vi "Generate Error.vi"(0 "Optional String":string, 1 "Class":refnum<class>, 2 "Error Code":i32, 3 "Error/Warning":bool=TRUE) -> (6 "error out":errorcluster)   [LabVIEW 2026, in "TALOS.lvlib"]
doc: "This VI generates the custom error, given its number. If the optional flag \"Error/Warning\" is set to False, a warning is generated. The optional String gets appended at the end of the error message.\nIf a Class is given in input, its name will also be added to the error string."
uses:
  TALOS.lvlib
  <vilib>/Utility/error.llb/DialogType.ctl
  Ancestor/Ancestor/Ancestor.lvclass
  Ancestor/Ancestor/Ancestor.lvclass/Ancestor.ctl
  FGV/Error Memory/Error Memory Core.vi
  <vilib>/AdvancedString/Delimited String to 1D String Array.vi
  <vilib>/AdvancedString/Delimited String to 1D String Array (string).vi
  Circus Root Path.vi
  FGV/Error Memory/Error Crt Lvl checker.vi
  FGV/Error Memory/Error Memory Core.vi/40c8088d-b597-4017-91af-faa98e00292e.vi
  FGV/Error Memory/Error Memory Core.vi/d4a3ab98-063c-4e44-b43d-fbdcfe6c2be2.vi
  Global Memory.vi
  <vilib>/Utility/LVClass/Get LV Class Name.vi
  Is in Packed Library.vi
  TALOS Root path.vi
  Read CSV worksheet.vi
  Global Constants.vi
  <vilib>/Comparison/Equal/Equal Functor/Equal Functor.lvclass
  FGV/Error Memory/Error Memory.lvlib
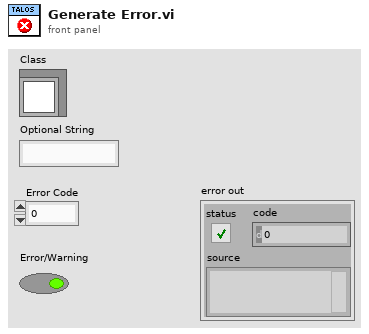
[diagram p1: front panel]
types:
  T1 = typedef "DialogType.ctl" = u16
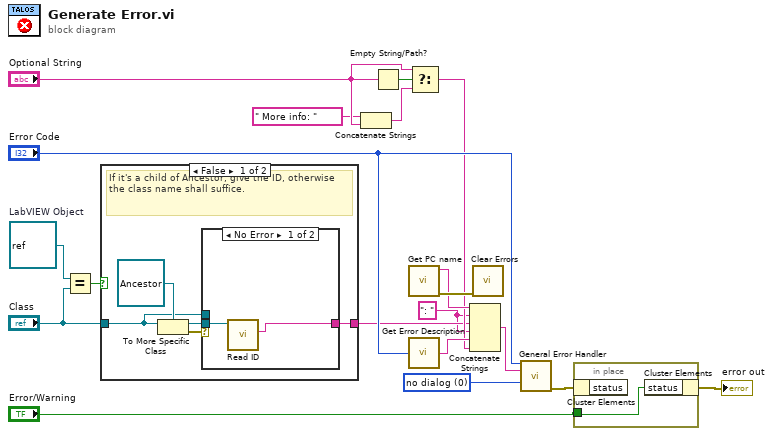
[diagram p0: block diagram]
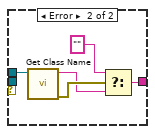
[diagram p2: hidden frame]
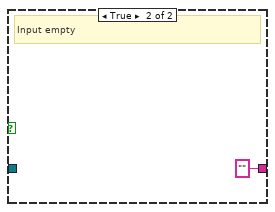
[diagram p3: hidden frame]
diagram:
  w3 = refnum<class> refnum  # LabVIEW Object
  w4 = ": " ("string")
  w18 = T1 0 items=["no dialog", "OK message", "continue or stop message", "OK message + warnings", "continue/stop + warnings"] ("type of dialog (OK msg:1)")
  n1 = Equal?(x=w3, y="Class") -> (x = y?=w1:bool)
  n2 = case shown="False" w1 {
    tunnel: [w24 "" ("Class Name")] -> w5
    tunnel: "Class" -> [w20 _]
    frame False {
      # "If it's a child of Ancestor, give the ID, otherwise the class name shall suffice."
      n3 = To More Specific Class(target class=refnum<class "Ancestor.lvclass"> refnum ("TALOS.lvlib:Ancestor.lvlib:Ancestor.lvclass"), reference=w20) -> (specific class reference=w22:refnum<class "Ancestor.lvclass">, error out=w21:errorcluster)  [unwired: 1 in]
      n4 = case shown="No Error" w21 {
        tunnel: [w25 w30] -> w24
        tunnel: w22 -> [w26 _]
        tunnel: w20 -> [_ w31]
        frame No Error {
          n5 = call "Read ID.vi"("Ancestor in"=w26) -> ("ID"=w25:string)  [unwired: 8 in, 2 out]
        }
        frame Error {
          n6 = call "Get Class Name.vi"("object"=w31) -> ("error out"=w29:errorcluster, "Class Name"=w28:string)  [unwired: 9 in]
          n7 = Select(t="", s=w29, f=w28) -> (s? t:f=w30:string)
        }
      }
    }
    frame True {
      # "Input empty"
    }
  }
  n8 = Concatenate Strings(" More info: " ("string"), "Optional String") -> (w8:string)
  n9 = Empty String/Path?(string/path="Optional String") -> (empty?=w10:bool)
  n10 = call "Get PC name.vi"() -> ("error out"=w19:errorcluster, "Hostname"=w11:string)  [unwired: 10 in]
  n11 = call "Get Error Description.vi"("Error Code in"="Error Code") -> ("Error Message out"=w17:string)  [unwired: 4 in]
  n12 = Select(t="Optional String", s=w10, f=w8) -> (s? t:f=w9:string)
  n13 = Concatenate Strings(w11, w4, w5, w4, w17, w9) -> (w12:string)
  n14 = call <vilib>:"Clear Errors.vi"("error in (no error)"=w19) -> ()  [unwired: 5 in, 2 out]
  n15 = call <vilib>:"General Error Handler.vi"("[error code] (0)"="Error Code", "[error source] (\" \")"=w12, "type of dialog (OK msg:1)"=w18) -> ("error out"=w15:errorcluster)  [unwired: 8 in, 4 out]
  n16 = in-place {
    in-place-border: "Error/Warning" -> [w33]
    n17 = in-place-cluster #1(w15) -> ()  [unwired: 1 out]
    n18 = in-place-cluster #1("status"=w33) -> (→"error out":errorcluster)
  }
